vi "FTW-EventLogger-AddRecord.vi"(0 "Event Logger":refnum<class "FTW-EventLogger-API.lvclass">, 5 "Event Type":string, 7 "Event Data":string, 9 "Source (unwired for call chain)":string="CallChain", 11 "Error to Log":errorcluster) -> (4 "Event Logger out":refnum<class "FTW-EventLogger-API.lvclass">, 6 "Serialized Event":string)   [LabVIEW 2013, in "FTW-EventLogger-API.lvclass"]
doc: "This method queues an event to be logged by the Logger associated with the LoggerID."
uses:
  FTW-EventLogger-API.lvclass
  FTW-EventLogger-API.lvclass/FTW-EventLogger-API.ctl
  Messaging/Messenger.Actor/FTW-Messenger-Actor.lvclass
panel:
  # "Inputs"
  # "Outputs"
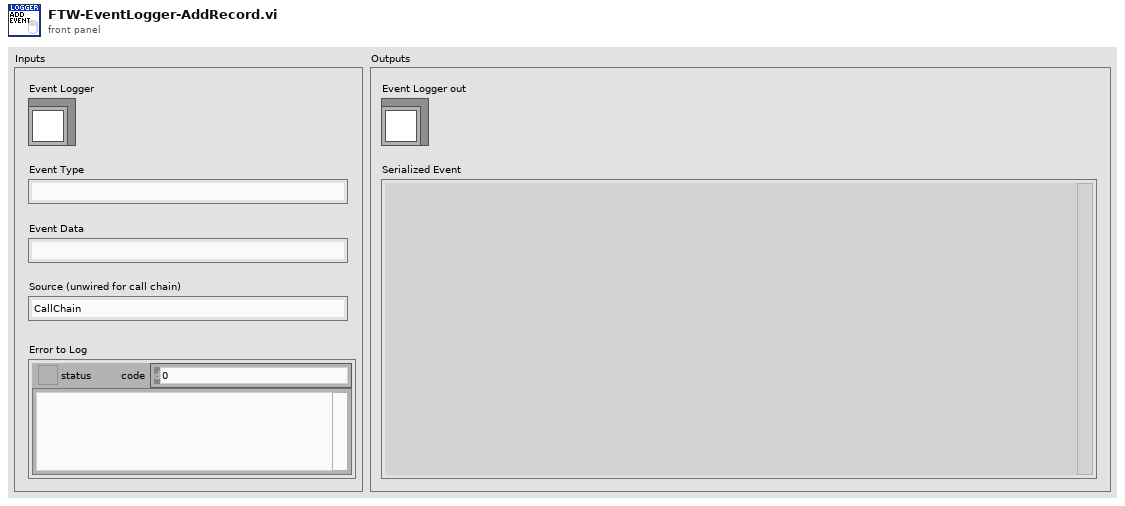
[diagram p1: front panel]
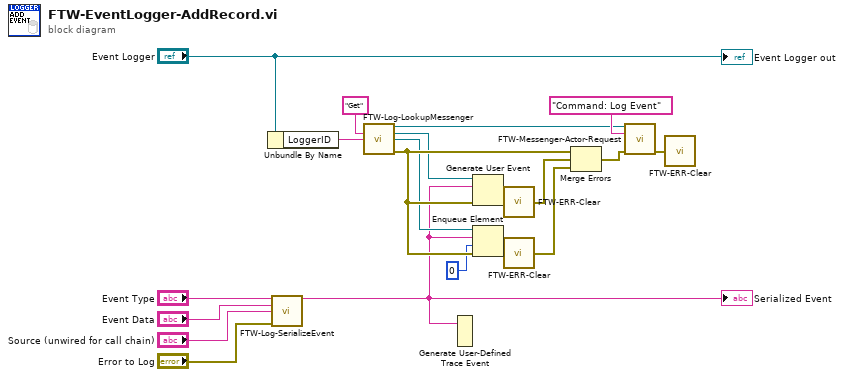
[diagram p0: block diagram]
diagram:
  n1 = Unbundle By Name("Event Logger") -> ("LoggerID"=w3:string)
  n2 = call "FTW-Log-SerializeEvent.vi"("Event Type"="Event Type", "Event Data"="Event Data", "Source (unwired for call chain, Empty to omit)"="Source (unwired for call chain)", "Error to Log"="Error to Log") -> ("Serialized Event"=w2:string)  [unwired: 11 in]
  "Serialized Event" <- w2
  n3 = call "FTW-Log-LookupMessenger.vi"("Action"="Get", "LoggerID"=w3) -> ("Logger Messenger out"=w6:refnum<class "FTW-Messenger-Actor.lvclass">, "Logged Event Broadcast"=w8:refnum<user-event>, "Log Queue"=w10:refnum<queue>, "error out"=w13:errorcluster)  [unwired: 10 in]
  n4 = Generate User-Defined Trace Event(2:w2) -> ()  [unwired: 1 in]
  n5 = Generate User Event(user event=w8, event data cluster=w2, error in=w13) -> (error out=w9:errorcluster)  [unwired: 1 in, 1 out]
  n6 = Enqueue Element(queue=w10, element=w2, timeout in ms (-1)=0, error in (no error)=w13) -> (error out=w11:errorcluster)  [unwired: 2 out]
  n7 = call "FTW-ERR-Clear.vi"("error to snuff"=w9) -> ("no error"=w15:errorcluster)
  n8 = call "FTW-ERR-Clear.vi"("error to snuff"=w11) -> ("no error"=w16:errorcluster)
  n9 = Merge Errors(w13, w15, w16) -> (w14:errorcluster)
  n10 = call-dynamic "FTW-Messenger-Actor-Request.vi"("Messenger"=w6, "Parameter"="Command: Log Event", "error in"=w14) -> ("error out"=w1:errorcluster)  [unwired: 11 in, 1 out]
  n11 = call "FTW-ERR-Clear.vi"("error to snuff"=w1) -> ()  [unwired: 1 out]
  "Event Logger out" <- "Event Logger"
